vi "Rampa_Pos&Neg.vi"(0 "task/channels in":refnum<k21>, 1 "Start_A":dbl caption="Ángulo inicial" min=-5.0 max=5.0 step=0.05, 2 "Stop_A":dbl caption="Ángulo final" min=-5.0 max=5.0 step=0.05, 3 "Step_A":dbl=0.01 caption="Paso ángulo" min=0.01 max=1.0 step=0.05, 4 "ms to wait":u32=20 min=7 max=1000 step=1, 5 "Error In":errorcluster) -> (19 "Error Out":errorcluster)   [LabVIEW 2016]
doc: "Decide que sub VI ejecutar dependiendo de los parametros \nde la rampá que se quiere ejecutar de +->- o de - ->+."
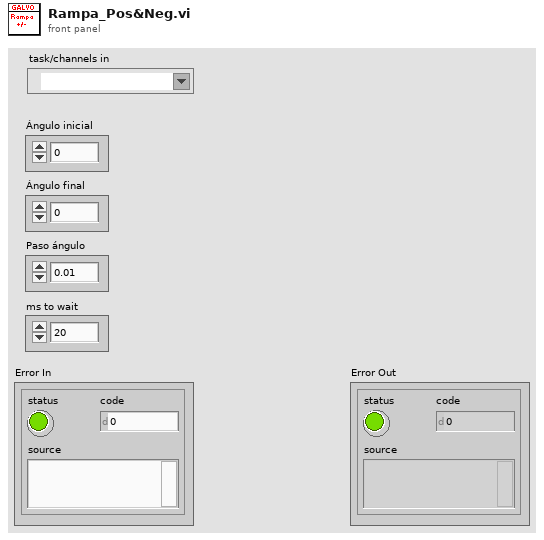
[diagram p1: front panel]
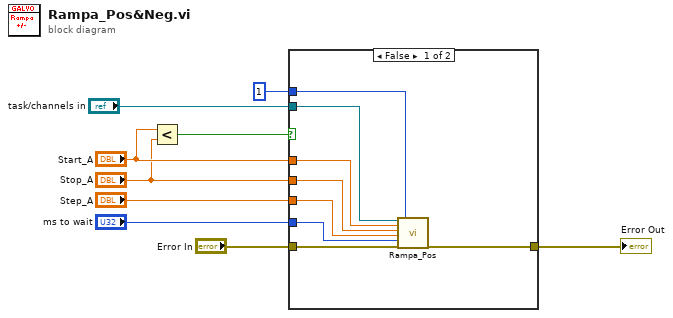
[diagram p0: block diagram]
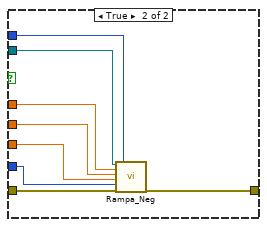
[diagram p2: hidden frame]
diagram:
  n1 = Less?(x="Start_A", y="Stop_A") -> (x < y?=w7:bool)
  n2 = case shown="False" w7 {
    tunnel: [w17 w25] -> w8
    tunnel: "Error In" -> [w16 w24]
    tunnel: u16 1 ("# Ciclos") -> [w10 w23]
    tunnel: "Start_A" -> [w15 w20]
    tunnel: "Stop_A" -> [w14 w19]
    tunnel: "Step_A" -> [w13 w18]
    tunnel: "ms to wait" -> [w12 w22]
    tunnel: "task/channels in" -> [w11 w21]
    frame False {
      n3 = call "Rampa_Pos.vi"("task/channels in"=w11, "Start_A"=w15, "Stop_A"=w14, "Step_A"=w13, "ms to wait"=w12, "Error In"=w16, "# Ciclos"=w10) -> ("Error Out"=w17:errorcluster)  [unwired: 12 in]
    }
    frame True {
      n4 = call "Rampa_Neg.vi"("task/channels in"=w21, "Start_A"=w20, "Stop_A"=w19, "Step_A"=w18, "ms to wait"=w22, "Error In"=w24, "# Ciclos"=w23) -> ("Error Out"=w25:errorcluster)  [unwired: 12 in]
    }
  }
  "Error Out" <- w8
